vi "IntakeQCP.vi"   [LabVIEW 2017]
uses:
  <userlib>/836-Library/System/QCP_V2/QCPSupportCode/QCP_GetDbl.vi
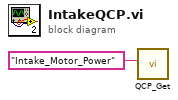
[diagram p0: block diagram]
diagram:
  n1 = call-poly <userlib>:"QCP_Get.vi"("Value Name"="Intake_Motor_Power") -> ()  [unwired: 8 in, 3 out]
